vi "Metric To Prometheus Lines.vi"(8 "error in (no error)":errorcluster, 10 "Include Metadata":bool=TRUE, 11 "Histograms.lvlib:Histogram.lvclass":refnum<class "Histogram.lvclass">) -> (0 "error out":errorcluster, 3 "Prometheus Lines":string[](array[string]))   [LabVIEW 2020, in "Metrics.lvlib" / "Histogram.lvclass"]
uses:
  Histogram.lvclass
  Histogram.lvclass/Histogram.ctl
  metric/Metric.lvclass
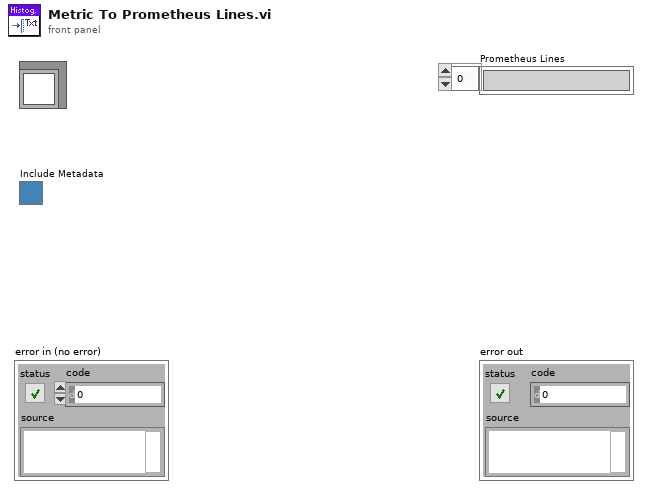
[diagram p1: front panel]
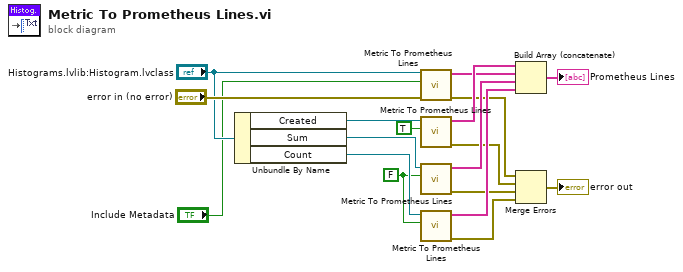
[diagram p0: block diagram]
diagram:
  w10 = FALSE ("Include Metadata")
  n1 = Unbundle By Name("Histograms.lvlib:Histogram.lvclass") -> ("Created"=w16:refnum<class "Metric.lvclass">, "Sum"=w12:refnum<class "Metric.lvclass">, "Count"=w11:refnum<class "Metric.lvclass">)
  n2 = call-parent "Metric To Prometheus Lines.vi"("error in (no error)"="error in (no error)", "Include Metadata"="Include Metadata", "Metrics.lvlib:Metric.lvclass"="Histograms.lvlib:Histogram.lvclass") -> ("error out"=w7:errorcluster, "Prometheus Lines"=w14:string[])  [unwired: 7 in]
  n3 = call-dynamic "Metric To Prometheus Lines.vi"("Include Metadata"=TRUE, "Metrics.lvlib:Metric.lvclass"=w16) -> ("error out"=w6:errorcluster, "Prometheus Lines"=w15:string[])  [unwired: 8 in]
  n4 = call-dynamic "Metric To Prometheus Lines.vi"("Include Metadata"=w10, "Metrics.lvlib:Metric.lvclass"=w12) -> ("error out"=w5:errorcluster, "Prometheus Lines"=w9:string[])  [unwired: 8 in]
  n5 = call-dynamic "Metric To Prometheus Lines.vi"("Include Metadata"=w10, "Metrics.lvlib:Metric.lvclass"=w11) -> ("error out"=w4:errorcluster, "Prometheus Lines"=w8:string[])  [unwired: 8 in]
  n6 = Build Array (concatenate)(w15, w14, w9, w8) -> (→"Prometheus Lines":string[])
  n7 = Merge Errors(w7, w6, w5, w4) -> (→"error out":errorcluster)
